vi "Write FlexLogger Data.vi"() -> ()   [LabVIEW 2024]
doc: "Demonstrates how to use network streams to pass data and commands between two running VIs. It displays waveform data that is received from the target VI and sends commands to update the frequency of the generated signal."
uses:
  <resource>/objmgr/ni.dex.rc
panel:
  out "Connected to reader":bool
  in  "stop":bool
  out "Data":waveform(dbl)[](graph)
  # "Overview: Demonstrates how to use Network Streams to write data to the FlexLogger StreamReader plug-in.\nRequirements: Windows\nInstructions:\n1. Run this VI.\n2. Add the StreamReader plug-in in FlexLogger.\n3. Configure the Reader using gear on right and set Writer URL to \"//localhost:labview/data/writer\".\n4. Press OK.\n5. When done, click Stop to stop the VI."
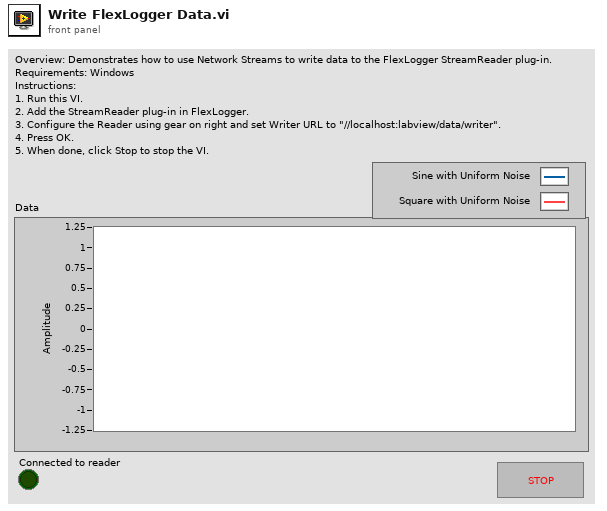
[diagram p1: front panel]
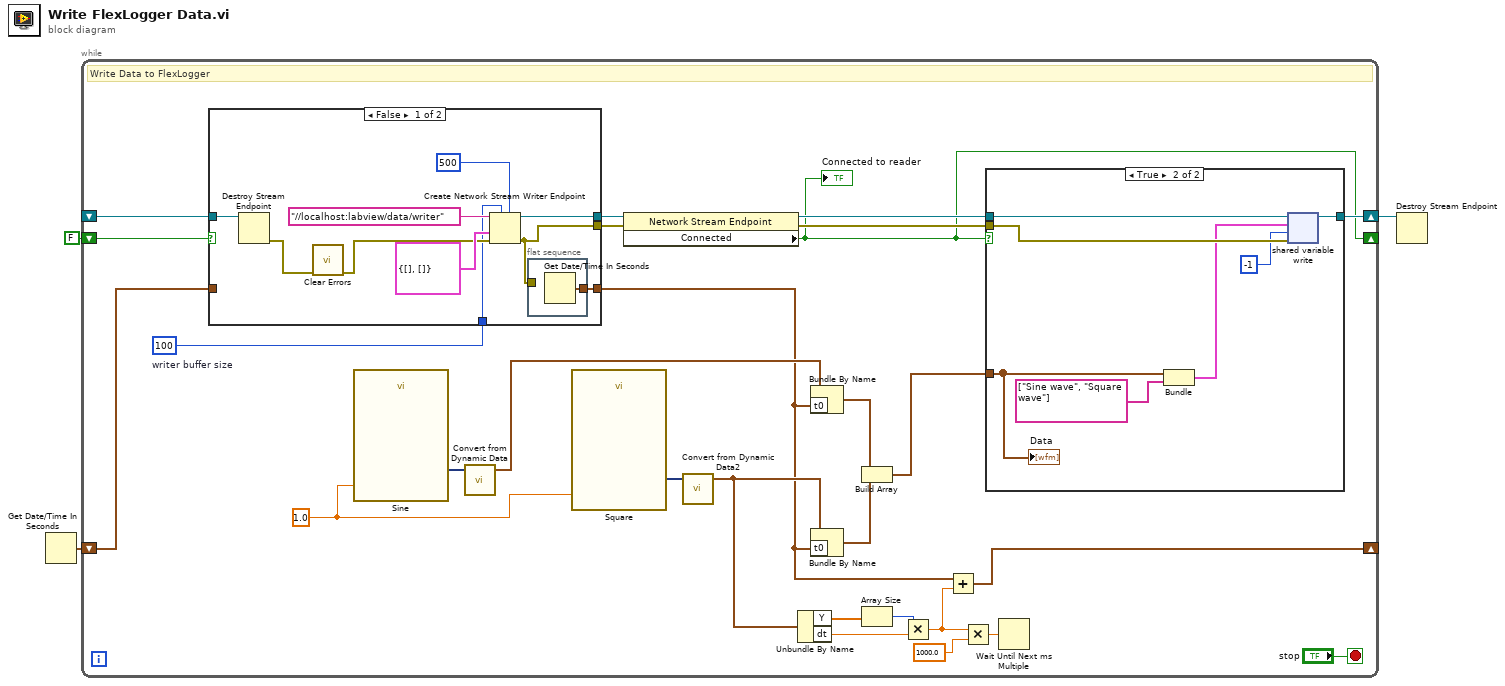
[diagram p0: block diagram]
diagram:
  n1 = Get Date/Time In Seconds() -> (seconds since 1Jan1904=w2:timestamp)
  n2 = while "Target->Host Data Reader" {
    shift-right: [w25] -> w3
    shift-left: _ -> [w24]
    shift-right: [w16] -> _
    shift-left: w2 -> [w4]
    shift-right: [w10] -> _
    shift-left: FALSE -> [w15]
    stop <- "stop" stop-if-true
    w9 = 100  # writer buffer size
    w28 = 1.0
    # "Write Data to FlexLogger"
    n3 = case shown="False" w15 {
      tunnel: [w32 _] -> w13
      tunnel: [w34 w43] -> w14
      tunnel: w24 -> [w37 w43]
      tunnel: w9 -> [w33 _]
      tunnel: [w31 w42] -> w5
      tunnel: w4 -> [_ w42]
      frame False {
        n4 = Destroy Stream Endpoint(11:w37) -> (0:w36:errorcluster)  [unwired: 1 in]
        n5 = call <vilib>:"Clear Errors.vi"("error in (no error)"=w36) -> ("error out"=w35:errorcluster)  [unwired: 5 in, 1 out]
        n6 = Create Network Stream Writer Endpoint(5:500 ("timeout in ms (-1)"), 7:w33, 8:w35, 9:cluster{waveform(dbl)[], string[]} {[], []} ("output cluster"), 11:"//localhost:labview/data/writer" ("writer name")) -> (0:w32:errorcluster, 3:w34:refnum<k21>)  [unwired: 2 in]
        n7 = flat-sequence {
          tunnel: w32 -> [_]
          tunnel: [w41] -> w31
          frame #0 {
            n8 = Get Date/Time In Seconds() -> (seconds since 1Jan1904=w41:timestamp)
          }
        }
      }
      frame True {
      }
    }
    n9 = call "Sine"("Frequency"=w28) -> ("Sine with Uniform Noise"=w29:dynamicdata)  [unwired: 13 in, 1 out]
    n10 = call "Convert from Dynamic Data"("Dynamic Data Type"=w29) -> ("Waveform"=w22:waveform(dbl))  [unwired: 3 in]
    n11 = call "Square"("Frequency"=w28) -> ("Square with Uniform Noise"=w30:dynamicdata)  [unwired: 13 in, 1 out]
    n12 = property class="Network Stream Endpoint"(reference=w14, error in=w13) -> (reference out=w11:refnum<k21>, error out=w12:errorcluster, "Connected"=w10:bool)
    "Connected to reader" <- w10
    n13 = call "Convert from Dynamic Data2"("Dynamic Data Type"=w30) -> ("Waveform"=w20:waveform(dbl))  [unwired: 3 in]
    n14 = Unbundle By Name(w20) -> ("Y"=w19:dbl[], "dt"=w17:dbl)
    n15 = Bundle By Name(cluster=w22, "t0"=w5) -> (w23:waveform(dbl))
    n16 = Bundle By Name(cluster=w20, "t0"=w5) -> (w21:waveform(dbl))
    n17 = Build Array(w23, w21) -> (w27:waveform(dbl)[])
    n18 = Array Size(array=w19) -> (size(s)=w18:i32)
    n19 = Multiply(x=w18, y=w17) -> (x*y=w8:dbl)
    n20 = Add(x=w5, y=w8) -> (x+y=w16:timestamp)
    n21 = Multiply(x=w8, y=1000.0) -> (x*y=w6:dbl)
    n22 = case shown="True" w10 {
      tunnel: w11 -> [w44 w51]
      tunnel: w12 -> [_ w50]
      tunnel: [w44 w49] -> w25
      tunnel: w27 -> [_ w45]
      frame False {
      }
      frame True {
        n23 = Bundle(w45, string[] ["Sine wave", "Square wave"]) -> (w47:cluster{waveform(dbl)[], string[]})  [unwired: 1 in]
        n24 = shared-variable-write(w51, w50, w47, -1 ("timeout ms (-1)")) -> (w49:refnum<k21>)  [unwired: 2 out]
        "Data" <- w45
      }
    }
    n25 = Wait Until Next ms Multiple(millisecond multiple=w6) -> ()  [unwired: 1 out]
  }
  n26 = Destroy Stream Endpoint(11:w3) -> ()  [unwired: 1 in, 1 out]
